vi "GetDiffFiles.vi"(8 "error in (no error)":errorcluster, 10 "Dest Files":path[](array[path]), 11 "Local Files":path[](array[path])) -> (0 "error out":errorcluster, 2 "DestToLocal":path[](array[path]), 3 "LocalToDest":path[](array[path]))   [LabVIEW 2022 SP3]
panel:
  out "DestToLocal Count":i32
  out "LocalToDest Count":i32
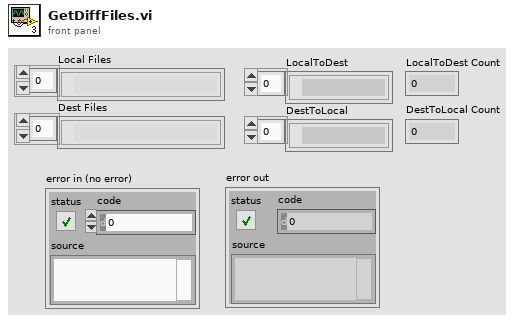
[diagram p1: front panel]
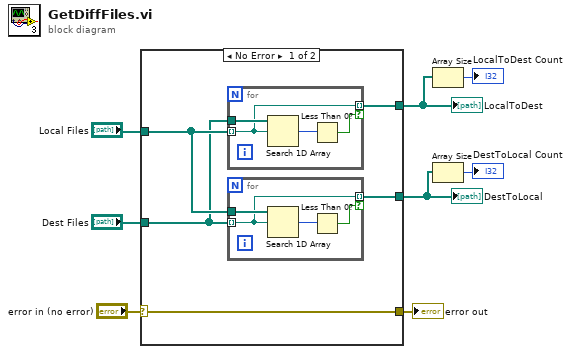
[diagram p0: block diagram]
diagram:
  n1 = case shown="No Error" "error in (no error)" {
    selector: "error in (no error)" -> [w13 w22]
    tunnel: [w13 w22] -> w7
    tunnel: "Dest Files" -> [w11 _]
    tunnel: "Local Files" -> [w12 _]
    tunnel: [w10 _] -> w4
    tunnel: [w9 _] -> w1
    frame No Error {
      n2 = for {
        tunnel: w12 -> [w16] mode=indexing
        tunnel: w11 -> [w17]
        tunnel: [w16] -> w10 mode=indexing if=w14
        n3 = Search 1D Array(1D array=w17, element=w16) -> (index of element=w15:i32)  [unwired: 1 in]
        n4 = Less Than 0?(x=w15) -> (x < 0?=w14:bool)
      }
      n5 = for {
        tunnel: w11 -> [w20] mode=indexing
        tunnel: w12 -> [w21]
        tunnel: [w20] -> w9 mode=indexing if=w18
        n6 = Search 1D Array(1D array=w21, element=w20) -> (index of element=w19:i32)  [unwired: 1 in]
        n7 = Less Than 0?(x=w19) -> (x < 0?=w18:bool)
      }
    }
    frame Error {
    }
  }
  "error out" <- w7
  "LocalToDest" <- w4
  "DestToLocal" <- w1
  n8 = Array Size(array=w4) -> (size(s)=→"LocalToDest Count":i32)
  n9 = Array Size(array=w1) -> (size(s)=→"DestToLocal Count":i32)
